vi "DatabaseInfoAdapter.vi"(8 "error in (no error)":errorcluster, 10 "recordset data":variant[][](array[variant]), 11 "UserBasicInfo":refnum<class "UserBasicInfo.lvclass">) -> (0 "error out":errorcluster, 2 "Result":string[][](array[string]), 3 "UserBasicInfo out":refnum<class "UserBasicInfo.lvclass">)   [LabVIEW 2015, in "UserManagement.lvlib" / "UserBasicInfo.lvclass"]
doc: "Adapter : <b> Convert database type to UI Type"
uses:
  UserManagement/UserBasicInfo/UserBasicInfo.lvclass
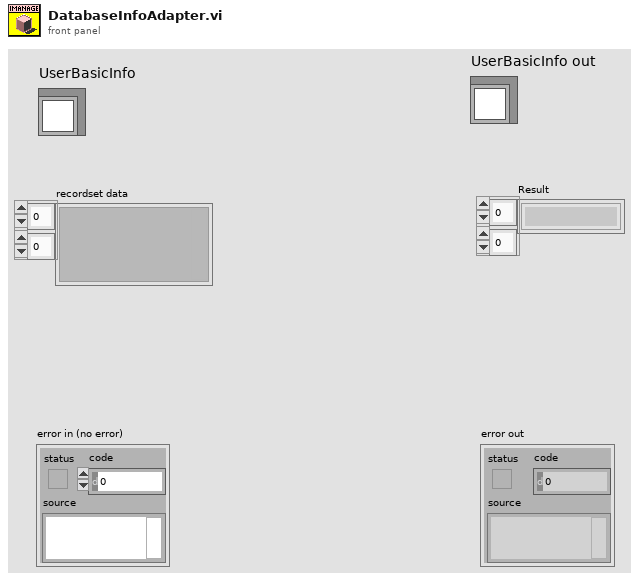
[diagram p1: front panel]
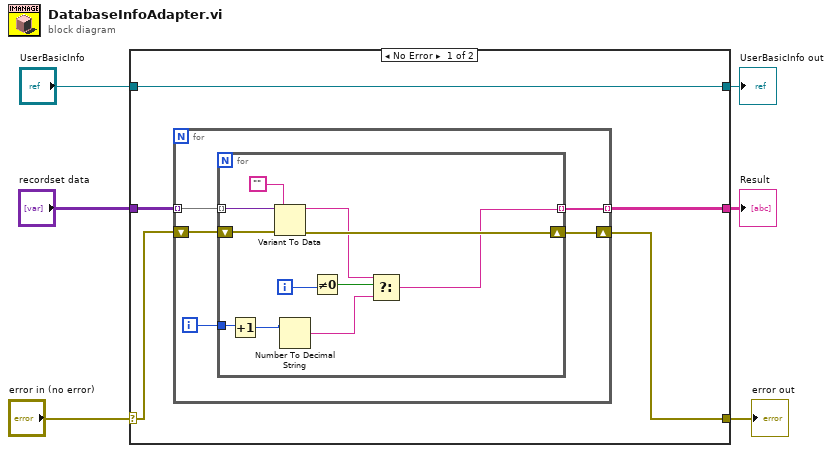
[diagram p0: block diagram]
diagram:
  n1 = case shown="No Error" "error in (no error)" {
    selector: "error in (no error)" -> [w10 w29]
    tunnel: [w9 w29] -> w5
    tunnel: "recordset data" -> [w11 _]
    tunnel: [w8 _] -> w3
    tunnel: "UserBasicInfo" -> [w7 w28]
    tunnel: [w7 w28] -> w1
    frame No Error {
      n2 = for {
        tunnel: w11 -> [w16] mode=indexing
        tunnel: [w15] -> w8 mode=indexing
        shift-right: [w13] -> w9
        shift-left: w10 -> [w14]
        i -> [w12]
        n3 = for {
          tunnel: w16 -> [w27] mode=indexing
          tunnel: [w17] -> w15 mode=indexing
          shift-right: [w24] -> w13
          shift-left: w14 -> [w25]
          tunnel: w12 -> [w20]
          i -> [w23]
          n4 = Increment(x=w20) -> (x+1=w19:i32)
          n5 = Variant To Data(error in=w25, type="", Variant=w27) -> (data=w21:string, error out=w24:errorcluster)
          n6 = Number To Decimal String(number=w19) -> (decimal integer string=w18:string)  [unwired: 1 in]
          n7 = Not Equal To 0?(x=w23) -> (x != 0?=w22:bool)
          n8 = Select(t=w21, s=w22, f=w18) -> (s? t:f=w17:string)
        }
      }
    }
    frame Error {
    }
  }
  "error out" <- w5
  "Result" <- w3
  "UserBasicInfo out" <- w1
